vi "IMAQdx Get Bayer Parameters for FPGA.vi"(8 "error in (no error)":errorcluster, 11 "IMAQdx Session In":T2) -> (0 "error out":errorcluster, 2 "Bayer Parameters":T1={"Pattern"=0, "Red Gain"=1.0, "Green Gain"=1.0, "Blue Gain"=1.0} {"Pattern" items=["GB", "GR", "BG", "RG"]}, 3 "IMAQdx Session Out":T2)   [LabVIEW 2020, in "NI_Vision_Acquisition_Software.lvlib"]
doc: "Queries the host machine for the Bayer algorithm, pattern, and the red, green and blue color gains used to create an image. Outputs a raw Bayer image with information about how to decode it on the FPGA target. Use this VI to produce a color image that the FPGA target can process."
uses:
  NI_Vision_Acquisition_Software.lvlib
  IMAQdx.ctl
  C:/Program Files (x86)/National Instruments/LabVIEW 2020/resource/objmgr/imaqdx.rc
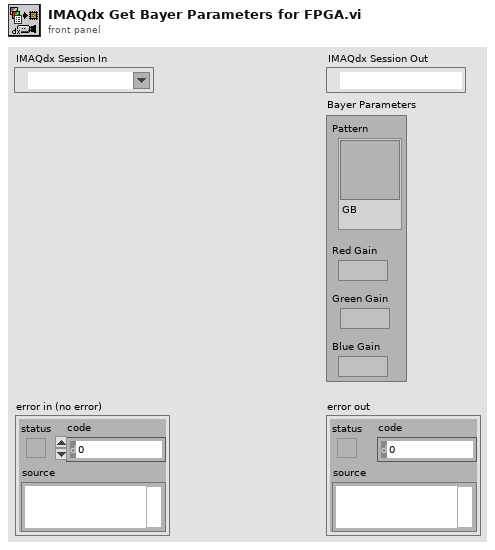
[diagram p1: front panel]
types:
  T1 = cluster{"Pattern":i32, "Red Gain":fxp<+,16,2>, "Green Gain":fxp<+,16,2>, "Blue Gain":fxp<+,16,2>}
  T2 = typedef "IMAQdx.ctl" = refnum<k21>
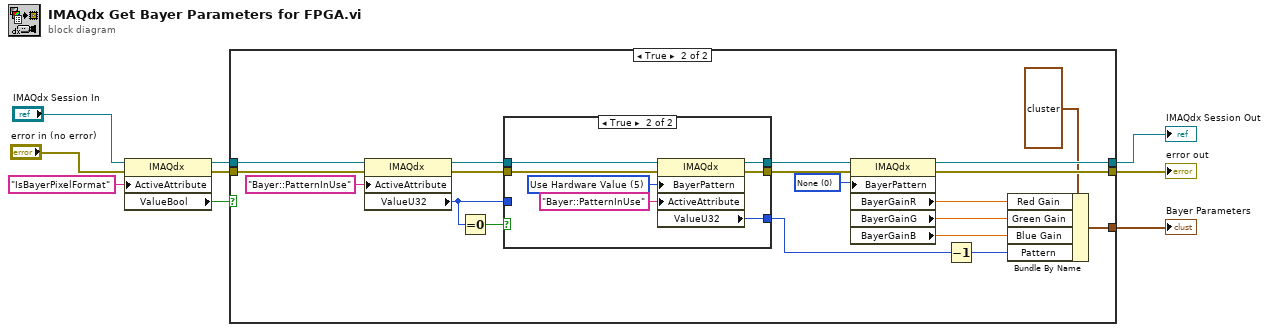
[diagram p0: block diagram]
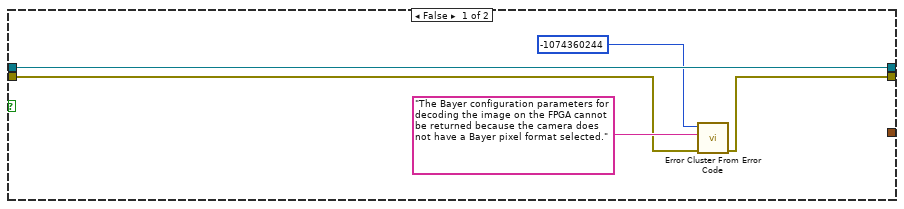
[diagram p2: hidden frame]
diagram:
  n1 = property class="IMAQdx"(reference="IMAQdx Session In", error in="error in (no error)", "ActiveAttribute"="IsBayerPixelFormat") -> (reference out=w7:T2, error out=w6:errorcluster, "ValueBool"=w5:bool)
  n2 = case shown="True" w5 {
    tunnel: w7 -> [w14 w33]
    tunnel: w6 -> [w11 w32]
    tunnel: [_ w18] -> w1
    tunnel: [w14 w17] -> w2
    tunnel: [w10 w16] -> w3
    frame False {
      n3 = call "Error Cluster From Error Code.vi"("error in (no error)"=w11, "error message (\"\")"="The Bayer configuration parameters for decoding the image on the FPGA cannot be returned because the camera does not have a Bayer pixel format selected." ("source"), "error code (0)"=-1074360244 ("code")) -> ("error out"=w10:errorcluster)  [unwired: 6 in]
    }
    frame True {
      w19 = u32 0 items=["None", "GB", "GR", "BG", "RG", "Use Hardware Value"] ("BayerPattern")
      n4 = property class="IMAQdx"(reference=w33, error in=w32, "ActiveAttribute"="Bayer::PatternInUse") -> (reference out=w30:T2, error out=w29:errorcluster, "ValueU32"=w27:u32)
      n5 = Equal To 0?(x=w27) -> (x = 0?=w28:bool)
      n6 = case shown="True" w28 {
        tunnel: w30 -> [w35 w43]
        tunnel: w29 -> [w34 w42]
        tunnel: w27 -> [w36 _]
        tunnel: [w36 w39] -> w21
        tunnel: [w35 w38] -> w25
        tunnel: [w34 w37] -> w26
        frame False {
        }
        frame True {
          w41 = u32 5 items=["None", "GB", "GR", "BG", "RG", "Use Hardware Value"] ("BayerPattern")
          n7 = property class="IMAQdx"(reference=w43, error in=w42, "BayerPattern"=w41, "ActiveAttribute"="Bayer::PatternInUse") -> (reference out=w38:T2, error out=w37:errorcluster, "ValueU32"=w39:u32)
        }
      }
      n8 = property class="IMAQdx"(reference=w25, error in=w26, "BayerPattern"=w19) -> (reference out=w17:T2, error out=w16:errorcluster, "BayerGainR"=w24:dbl, "BayerGainG"=w23:dbl, "BayerGainB"=w22:dbl)
      n9 = Decrement(x=w21) -> (x-1=w20:u32)
      n10 = Bundle By Name(cluster=T1 {"Pattern"=0, "Red Gain"=1.0, "Green Gain"=1.0, "Blue Gain"=1.0} ("Bayer Parameters"), "Red Gain"=w24, "Green Gain"=w23, "Blue Gain"=w22, "Pattern"=w20) -> (w18:T1)
    }
  }
  "error out" <- w3
  "IMAQdx Session Out" <- w2
  "Bayer Parameters" <- w1
